vi "CoMP-S Verify Observer Name.vi"(7 "Observer Programm":u16(ring) items=["OBS_PROG SELECTION", "TEST", "OBS_PROG 001: SPECTROPOLARIMETRY OF A QUIESCENT PROMINENCE AND ITS CAVITY", "OBS_PROG 002: SPECTROPOLARIMETRY OF TORNADOES IN LINE H ALPHA", "CAL_PROG 001: CORONAGRAPH FOCUS DETERMINATION FOR ALL LINES", "TEST_PROG 001: DATA ACQUISITION BY CAMERAS"], 9 "Observer 2":u16(ring) items=["Unknown", "INY", "RYBAK", "MACURA", "KOZAK", "KAVKA", "HABAJ", "AMBROZ"], 11 "Stop Button":bool) -> (0 "Out Stop":bool, 2 "Obs Selection":string="Select the OBSERVER NAME!", 3 "Observer Selection":bool)   [LabVIEW 2014]
panel:
  out "Prog Selection":string="Program selected"
  out "Program Selection":bool
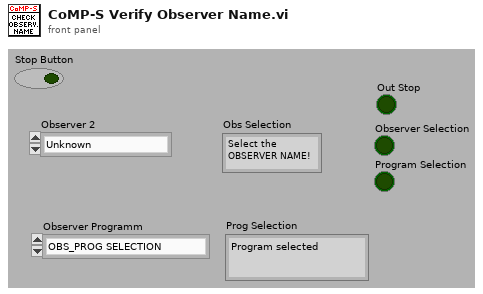
[diagram p1: front panel]
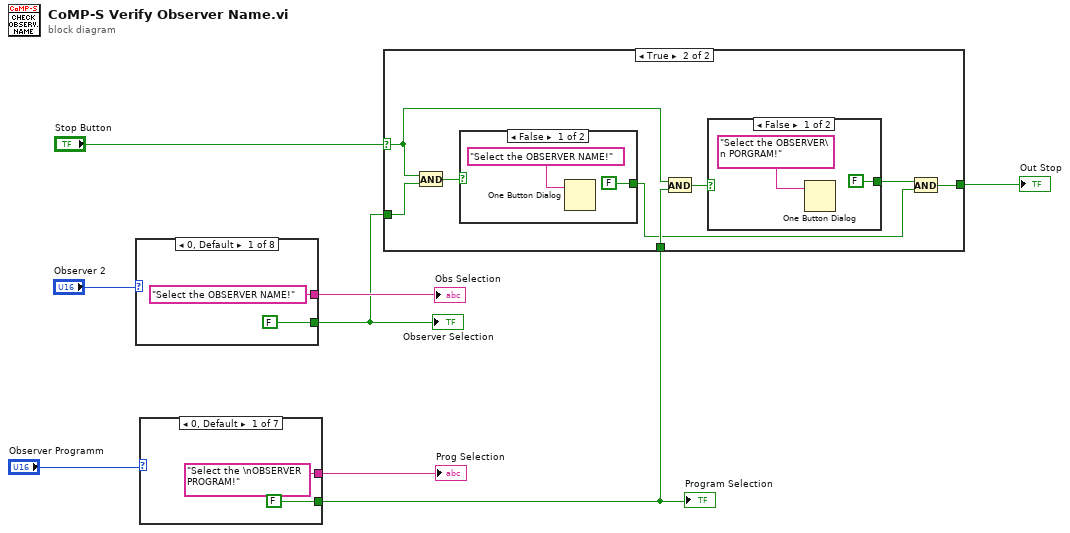
[diagram p0: block diagram]
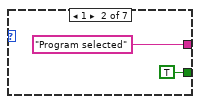
[diagram p2: hidden frame]
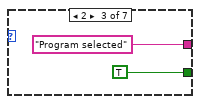
[diagram p3: hidden frame]
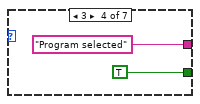
[diagram p4: hidden frame]
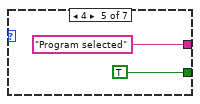
[diagram p5: hidden frame]
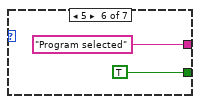
[diagram p6: hidden frame]
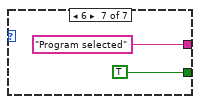
[diagram p7: hidden frame]
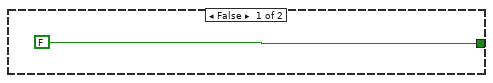
[diagram p8: hidden frame]
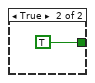
[diagram p9: hidden frame]
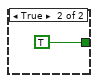
[diagram p10: hidden frame]
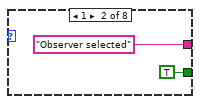
[diagram p11: hidden frame]
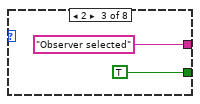
[diagram p12: hidden frame]
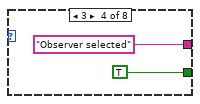
[diagram p13: hidden frame]
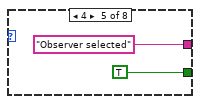
[diagram p14: hidden frame]
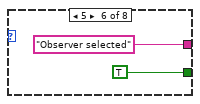
[diagram p15: hidden frame]
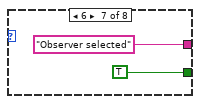
[diagram p16: hidden frame]
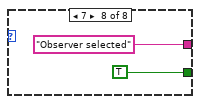
[diagram p17: hidden frame]
diagram:
  n1 = case shown="0, Default" "Observer 2" {
    tunnel: ["Select the OBSERVER NAME!" "Observer selected" "Observer selected" "Observer selected" "Observer selected" "Observer selected" "Observer selected" "Observer selected"] -> w8
    tunnel: [FALSE TRUE TRUE TRUE TRUE TRUE TRUE TRUE] -> w5
    frame 0, Default {
    }
    frame 1 {
    }
    frame 2 {
    }
    frame 3 {
    }
    frame 4 {
    }
    frame 5 {
    }
    frame 6 {
    }
    frame 7 {
    }
  }
  "Obs Selection" <- w8
  "Observer Selection" <- w5
  n2 = case shown="0, Default" "Observer Programm" {
    tunnel: ["Select the \nOBSERVER PROGRAM!" "Program selected" "Program selected" "Program selected" "Program selected" "Program selected" "Program selected"] -> w1
    tunnel: [FALSE TRUE TRUE TRUE TRUE TRUE TRUE] -> w2
    frame 0, Default {
    }
    frame 1 {
    }
    frame 2 {
    }
    frame 3 {
    }
    frame 4 {
    }
    frame 5 {
    }
    frame 6 {
    }
  }
  "Program Selection" <- w2
  "Prog Selection" <- w1
  n3 = case shown="True" "Stop Button" {
    selector: "Stop Button" -> [_ w43]
    tunnel: w5 -> [_ w47]
    tunnel: [FALSE w41] -> w4
    tunnel: w2 -> [_ w44]
    frame False {
    }
    frame True {
      n4 = And(x=w43, y=w47) -> (x .and. y?=w46:bool)
      n5 = case shown="False" w46 {
        tunnel: [FALSE TRUE] -> w40
        frame False {
          n6 = One Button Dialog(message="Select the OBSERVER NAME!") -> ()  [unwired: 1 in, 1 out]
        }
        frame True {
        }
      }
      n7 = And(x=w43, y=w44) -> (x .and. y?=w45:bool)
      n8 = case shown="False" w45 {
        tunnel: [FALSE TRUE] -> w42
        frame False {
          n9 = One Button Dialog(message="Select the OBSERVER\n PORGRAM!") -> ()  [unwired: 1 in, 1 out]
        }
        frame True {
        }
      }
      n10 = And(x=w42, y=w40) -> (x .and. y?=w41:bool)
    }
  }
  "Out Stop" <- w4
